vi "GetJoystickValues.vi"(11 "Jockstick Ref":string="Joystick 0") -> (1 "Joystick cluster":T1)   [LabVIEW 2019]
uses:
  <vilib>/Rock Robotics/WPI/Utilities/WPI_GetSetVariantRefNum.vi
panel:
  out "5":bool
  out "11":bool
  out "10":bool
  out "9":bool
  out "Button 3":bool
  out "Trigger":bool
  out "Rotation":dbl
  out "12":bool
  out "8":bool
  out "7":bool
  out "6":bool
  out "4":bool
  out "Side button":bool
  out "X-Axis":dbl(slide) scale=-1.0..1.0
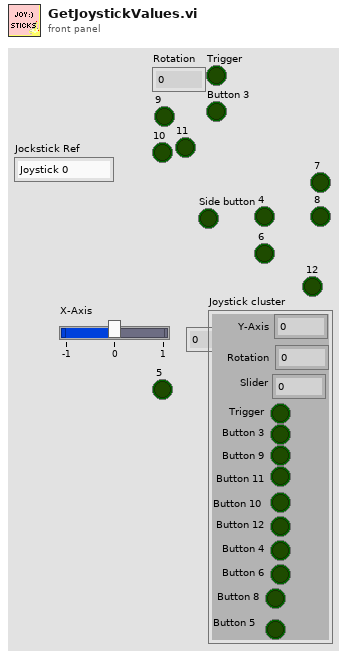
[diagram p1: front panel]
types:
  T1 = cluster{"Y-Axis":dbl, "Rotation":dbl, "Slider":dbl, "Trigger":bool, "Button 3":bool, "Button 9":bool, "Button 11":bool, "Button 10":bool, "Button 12":bool, "Button 4":bool, "Button 6":bool, "Button 8":bool, "Button 5":bool}
  T2 = typedef "WPI_JoystickDevRef.ctl" = cluster{"Device":T3}
  T3 = typedef "WPI_JoystickDeviceEnum.ctl" = enum16{"USB 0", "USB 1", "USB 2", "USB 3", "USB 4", "USB 5"}
  T4 = cluster{dbl, dbl, dbl, bool, bool, bool, bool, bool, bool, bool, bool, bool, bool}
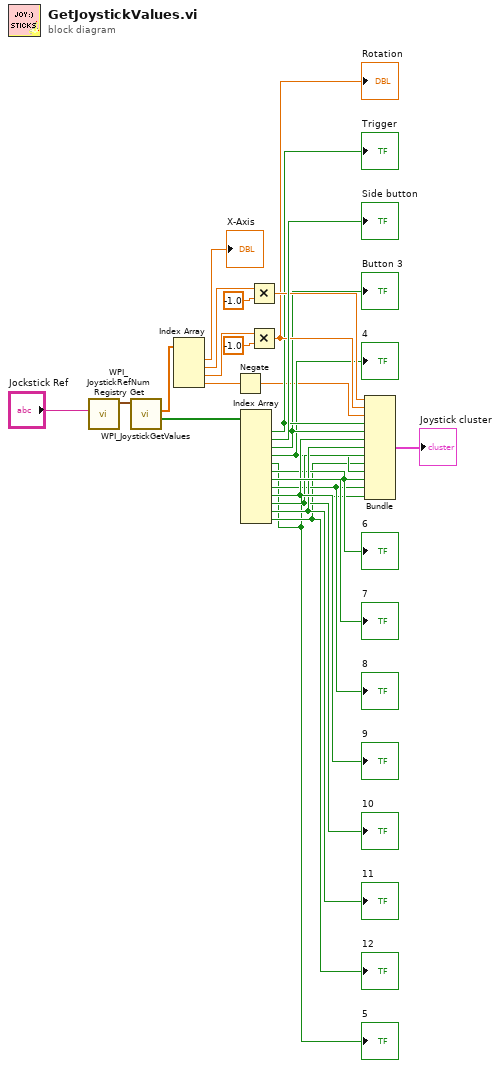
[diagram p0: block diagram]
diagram:
  n1 = call <vilib>:"WPI_JoystickRefNum Registry Get.vi"("refnum name"="Jockstick Ref") -> ("JoystickDevRef"=w26:T2)  [unwired: 9 in, 1 out]
  n2 = call <vilib>:"WPI_JoystickGetValues.vi"("JoystickDevRef"=w26) -> ("Buttons"=w24:bool[], "Axes"=w25:dbl[])  [unwired: 6 in, 3 out]
  n3 = Index Array(array=w25) -> (element #1=→"X-Axis":dbl, element #2=w20:dbl, element #3=w18:dbl, element #4=w13:dbl)  [unwired: 4 in]
  n4 = Negate(x=w13) -> (-x=w3:dbl)
  n5 = Index Array(array=w24) -> (element #1=w12:bool, element #2=→"Side button":bool, element #3=w11:bool, element #4=w6:bool, element #5=w1:bool, element #6=w5:bool, element #7=→"7":bool, element #8=w4:bool, element #9=w10:bool, element #10=w7:bool, element #11=w8:bool, element #12=w2:bool)  [unwired: 12 in]
  "4" <- w6
  "6" <- w5
  "8" <- w4
  "12" <- w2
  "Trigger" <- w12
  "Button 3" <- w11
  "9" <- w10
  "10" <- w7
  "11" <- w8
  "5" <- w1
  n6 = Multiply(x=w20, y=-1.0) -> (x*y=w15:dbl)
  n7 = Multiply(x=w18, y=-1.0) -> (x*y=w14:dbl)
  "Rotation" <- w14
  n8 = Bundle(w15, w14, w3, w12, w11, w10, w8, w7, w2, w6, w5, w4, w1) -> (→"Joystick cluster":T4)  [unwired: 1 in]
